vi "Write Battery Switch.vi"(8 "error in (no error)":errorcluster, 10 "Battery Switch Engine Refs in":T1 {"RT IDs"."Slot #" max=15; "RT IDs"."Chip Address (A2 A1 A0)" max=7; "RT Block Data Refs"."Data Reference" format="%.0x"}, 11 "DMA FIFO Ref in":refnum<k20>) -> (0 "error out":errorcluster, 2 "Battery Switch Engine Refs out":T1 {"RT IDs"."Slot #" max=15; "RT IDs"."Chip Address (A2 A1 A0)" max=7; "RT Block Data Refs"."Data Reference" format="%.0x"})   [LabVIEW 2014, in "SLSC configuration Engine.lvlib"]
uses:
  SLSC configuration Engine.lvlib
  Type Defs/RT Engine Refs.ctl
  Shared/Type Defs/RT IDs.ctl
  Shared/SPI Utility/Slot #.ctl
  Shared/MCP23S17/Chip Address.ctl
  <vilib>/NI Veristand/Custom Device API/Block Data Reference.ctl
  <vilib>/NI Veristand/Custom Device API/Data Reference.ctl
  <vilib>/NI Veristand/Custom Device API/Global Data Refs.vi
  Shared/Constants.vi
  <vilib>/NI Veristand/Custom Device API/Custom Device API.lvlib
  Shared/SLSC configuration Shared.lvlib
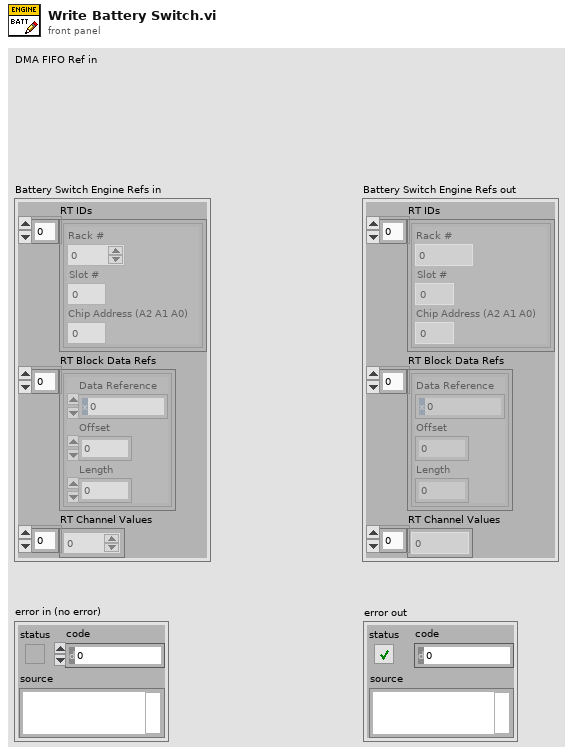
[diagram p1: front panel]
types:
  T1 = typedef "SLSC configuration Engine.lvlib/RT Engine Refs.ctl" = cluster{"RT IDs":T2[], "RT Block Data Refs":T5[], "RT Channel Values":dbl[]}
  T2 = typedef "SLSC configuration Shared.lvlib/RT IDs.ctl" = cluster{"Rack #":u8, "Slot #":T3, "Chip Address (A2 A1 A0)":T4}
  T3 = typedef "SLSC configuration Shared.lvlib/Slot #.ctl" = u8
  T4 = typedef "SLSC configuration Shared.lvlib/Chip Address.ctl" = u8
  T5 = typedef "Custom Device API.lvlib/Block Data Reference.ctl" = cluster{"Data Reference":T6, "Offset":i32, "Length":i32}
  T6 = typedef "Custom Device API.lvlib/Data Reference.ctl" = i32
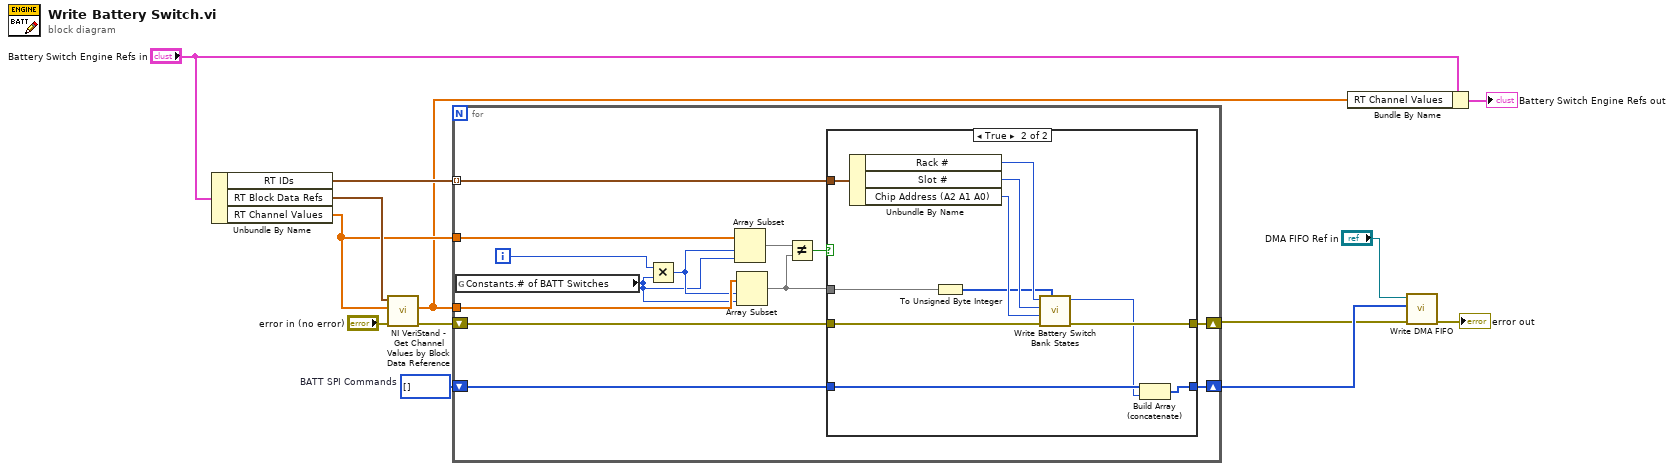
[diagram p0: block diagram]
diagram:
  w5 = u64[] []  # BATT SPI Commands
  n1 = Unbundle By Name("Battery Switch Engine Refs in") -> ("RT IDs"=w10:T2[], "RT Block Data Refs"=w13:T5[], "RT Channel Values"=w8:dbl[])
  n2 = call <vilib>:"NI VeriStand - Get Channel Values by Block Data Reference.vi"("error in (no error)"="error in (no error)", "Values Array in"=w8, "Block Data Ref"=w13) -> ("error out"=w11:errorcluster, "Values Array out"=w7:dbl[])  [unwired: 6 in, 1 out]
  n3 = for {
    shift-right: [w18] -> w2
    shift-left: w11 -> [w20]
    tunnel: w10 -> [w21] mode=indexing
    tunnel: w7 -> [w24]
    tunnel: w8 -> [w25]
    shift-right: [w15] -> w3
    shift-left: w5 -> [w16]
    i -> [w26]
    n4 = global read "Constants.vi" "Constants.# of BATT Switches"() -> (w14:u8)
    n5 = Multiply(x=w26, y=w14) -> (x*y=w23:i32)
    n6 = Array Subset(array=w25, index=w23, length=w14) -> (w22:dbl[])
    n7 = Array Subset(array=w24, index=w23, length=w14) -> (w19:dbl[])
    n8 = Not Equal?(x=w22, y=w19) -> (x != y?=w17:bool)
    n9 = case shown="True" w17 {
      tunnel: w21 -> [_ w39]
      tunnel: w20 -> [w28 w38]
      tunnel: w19 -> [_ w34]
      tunnel: [w28 w32] -> w18
      tunnel: w16 -> [w27 w31]
      tunnel: [w27 w29] -> w15
      frame False {
      }
      frame True {
        n10 = Unbundle By Name(w39) -> ("Rack #"=w37:u8, "Slot #"=w36:T3, "Chip Address (A2 A1 A0)"=w35:T4)
        n11 = To Unsigned Byte Integer(number=w34) -> (unsigned 8bit integer=w33:u8[])
        n12 = call "Write Battery Switch Bank States.vi"("Battery Switch States"=w33, "error in (no error)"=w38, "Chip Address (A2 A1 A0)"=w35, "Slot #"=w36, "Rack #"=w37) -> ("error out"=w32:errorcluster, "FIFO SPI Message"=w30:u64)  [unwired: 4 in, 1 out]
        n13 = Build Array (concatenate)(w31, w30) -> (w29:u64[])
      }
    }
  }
  n14 = Bundle By Name(cluster="Battery Switch Engine Refs in", "RT Channel Values"=w7) -> (→"Battery Switch Engine Refs out":T1)
  n15 = call "Write DMA FIFO.vi"("error in (no error)"=w2, "FIU SPI Commands"=w3, "DMA FIFO Ref in"="DMA FIFO Ref in") -> ("error out"=→"error out":errorcluster)  [unwired: 8 in]
